vi "Kundt impulse.vi"() -> ()   [LabVIEW 2014]
uses:
  <vilib>/Analysis/2dsp.llb/Real FFT.vi
  <vilib>/Analysis/NI_AALPro.lvlib
panel:
  out "Waveform Graph":dbl[](graph)
  out "Averaged Signal":dbl[](graph)
  in  "number of samples":i32=100
  in  "Rate (Hz)":dbl
  in  "Averages":dbl
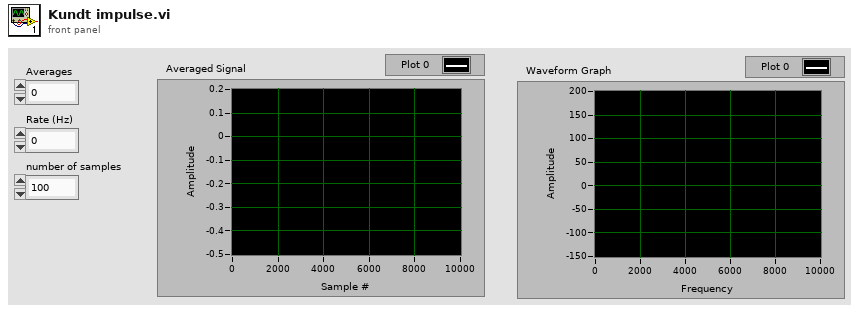
[diagram p1: front panel]
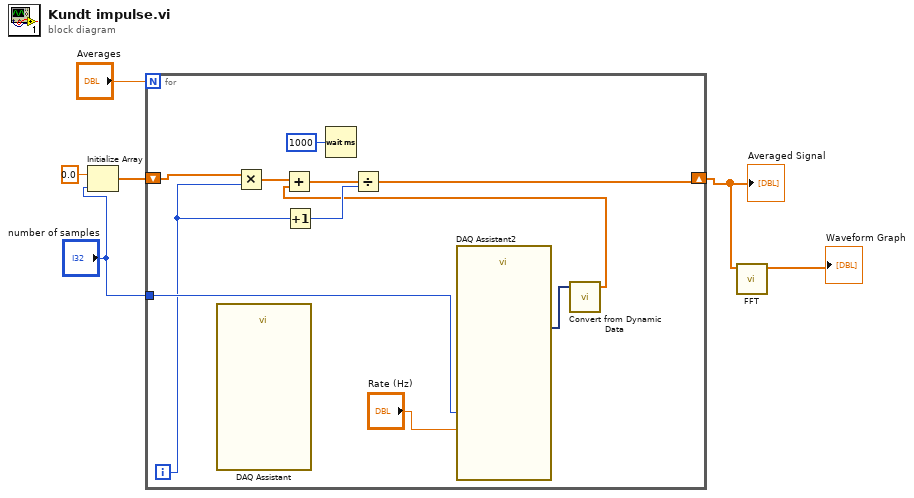
[diagram p0: block diagram]
diagram:
  n1 = Initialize Array(0.0 ("element"), "number of samples") -> (w3:dbl[])
  n2 = for {
    N: "Averages" -> [_]
    tunnel: "number of samples" -> [w15]
    shift-right: [w7] -> w2
    shift-left: w3 -> [w12]
    i -> [w11]
    n3 = call "DAQ Assistant"() -> ()  [unwired: 18 in, 2 out]
    n4 = Multiply(x=w12, y=w11) -> (x*y=w13:dbl[])
    n5 = Increment(x=w11) -> (x+1=w14:i32)
    n6 = Wait (ms)(milliseconds to wait=u32 1000) -> ()  [unwired: 1 out]
    n7 = call "DAQ Assistant2"("rate"="Rate (Hz)", "number of samples"=w15) -> ("data"=w10:dynamicdata)  [unwired: 15 in, 2 out]
    n8 = call "Convert from Dynamic Data"("Dynamic Data Type"=w10) -> ("Array"=w8:dbl[])  [unwired: 3 in]
    n9 = Add(x=w13, y=w8) -> (x+y=w9:dbl[])
    n10 = Divide(x=w9, y=w14) -> (x/y=w7:dbl[])
  }
  "Averaged Signal" <- w2
  n11 = call-poly <vilib>:"FFT.vi"("X"=w2) -> ("FFT {X}"=→"Waveform Graph":cdb[])  [unwired: 9 in, 1 out]
